vi "ground_station_control_only.vi"() -> ()   [LabVIEW 2017]
uses:
  <vilib>/Analysis/coordinate.llb/3D Cartesian Coordinate Rotation (Euler) (Array).vi
  <vilib>/Instr/_visa.llb/VISA Configure Serial Port (Instr).vi
  <vilib>/Analysis/NI_AALPro.lvlib
panel:
  out "read buffer":string
  in  "ZXZ":cluster{"phi":dbl, "theta":dbl, "psi":dbl} {"psi" min=0.0 max=6.28 step=0.01 format="%.2f"; "theta" min=0.0 max=3.14 step=0.01 format="%.2f"; "phi" min=0.0 max=6.28 step=0.001 format="%.2f"}
  out "时间差":u32 format="时间差 %.0f ms"
  out "外层":i32 format="外层循环 %.0f"
  out "String 4":string
  out "String 3":string
  in  "停止外层":bool
  out "Array":cluster{i32, i32, "read buffer":string}[](array[cluster])
  out "实际读取字节数":u32 format="实际读取的字节数 %.0f"
  out "内层":i32 format="内层循环 %.0f"
  in  "Z-":bool
  in  "Z+":bool
  in  "Y-":bool
  in  "Y+":bool
  in  "X-":bool
  in  "X+":bool
  out "error out 2":errorcluster
  out "String 2":string
  in  "Boolean":bool
  in  "VISA resource name":refnum<visa-resource-name>
  out "length":i32
  out "String":string
  out "error out":errorcluster
  in  "停止内层":bool
  in  "目标取向":dbl[][](array[numeric])
  in  "目标位置":dbl[](array[numeric]) step=0.1 format="%.1f"
  out "求解状态":i32
  out "关节角度":dbl[](array[numeric])
  in  "初始关节位置":dbl[][](array[numeric])
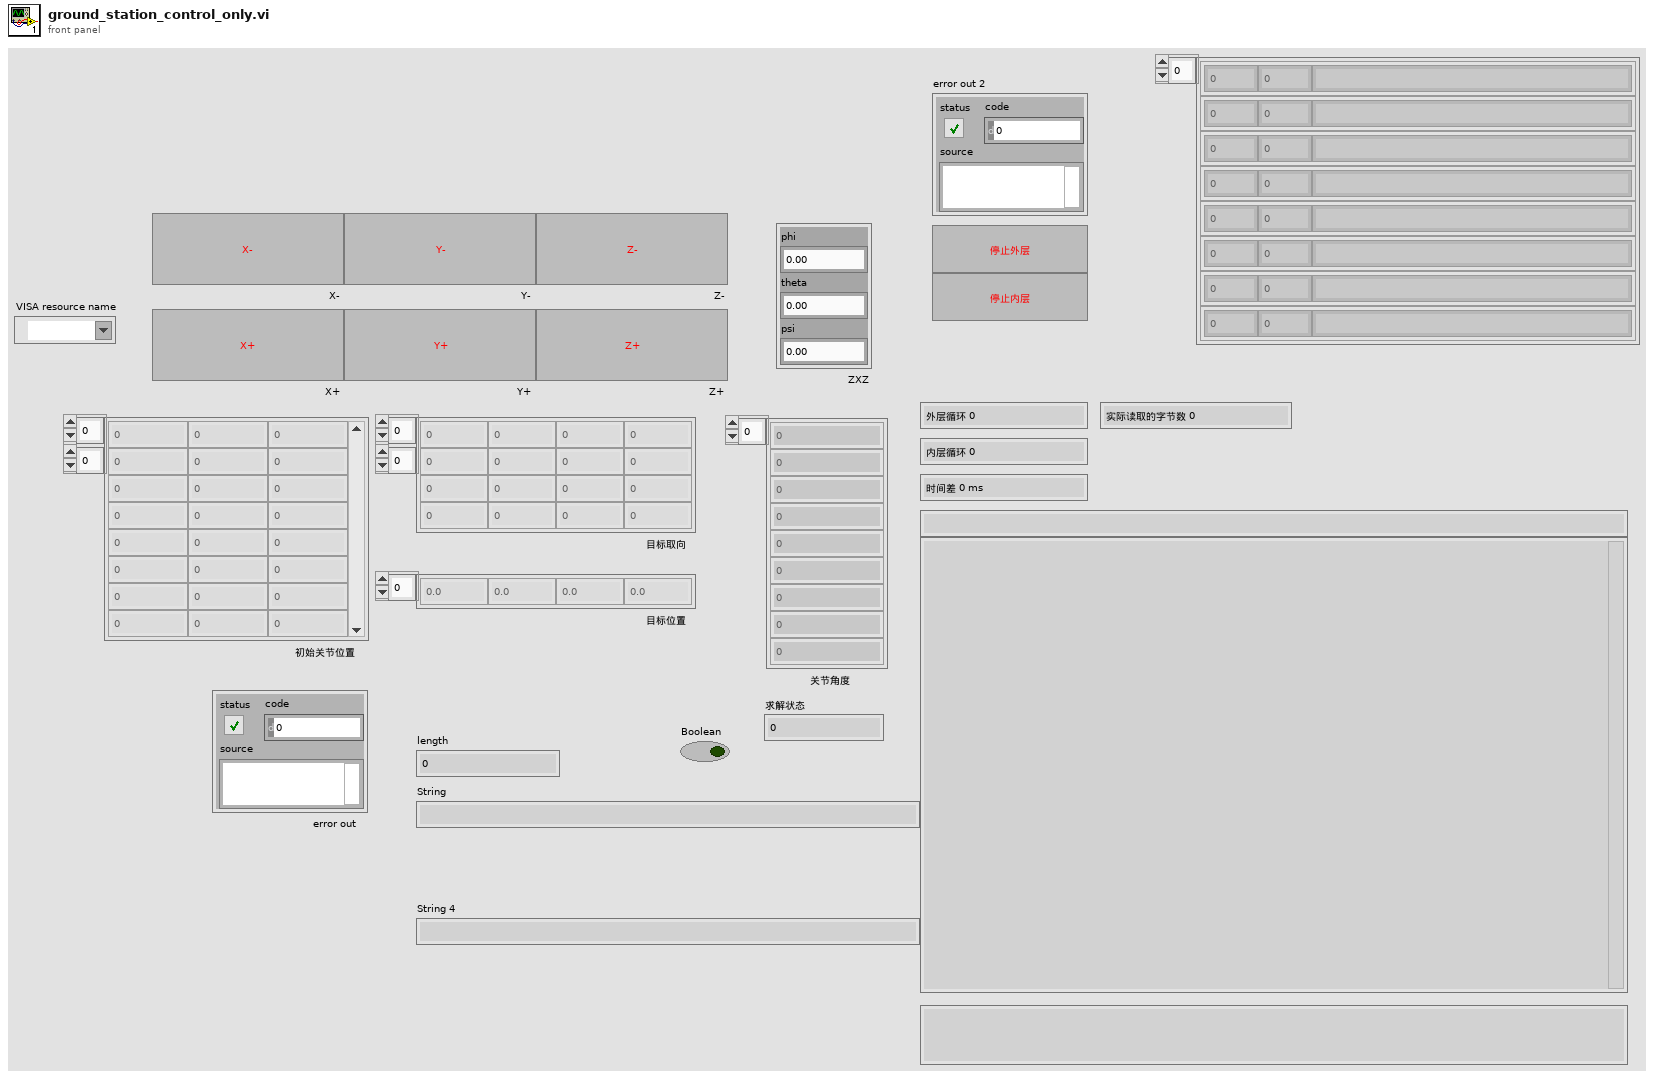
[diagram p1: front panel]
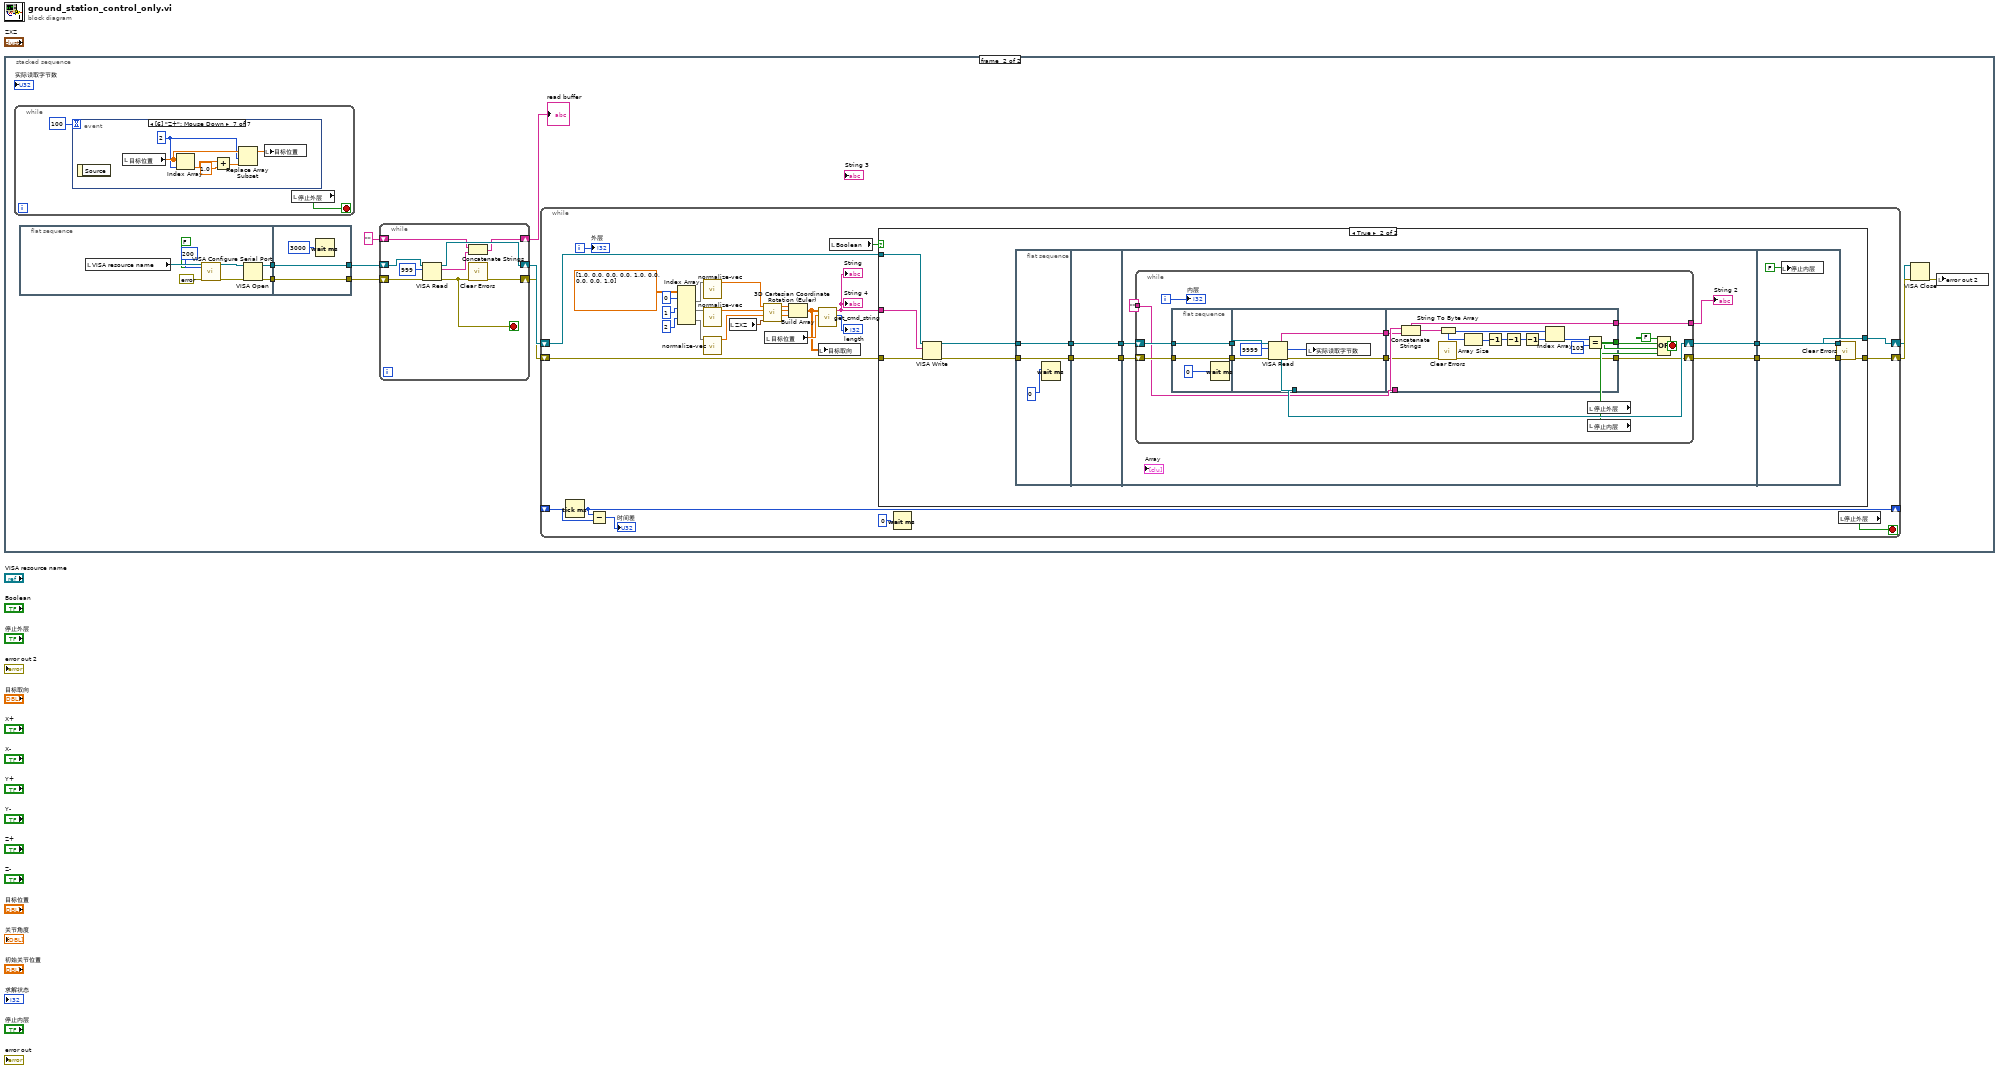
[diagram p0: block diagram]
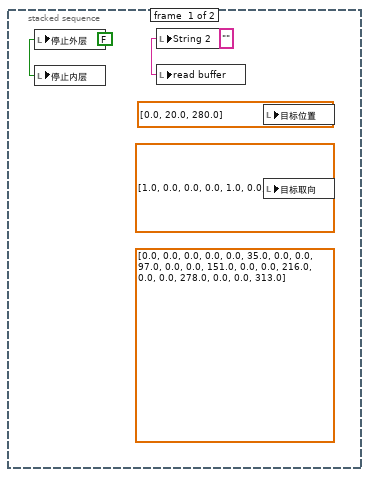
[diagram p2: hidden frame]
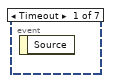
[diagram p4: hidden frame]
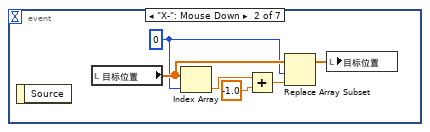
[diagram p5: hidden frame]
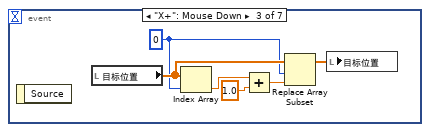
[diagram p6: hidden frame]
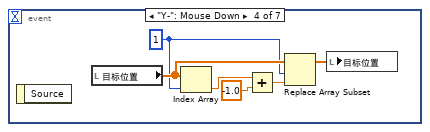
[diagram p7: hidden frame]
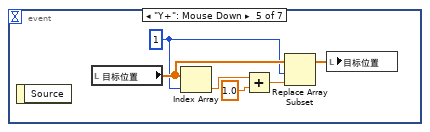
[diagram p8: hidden frame]
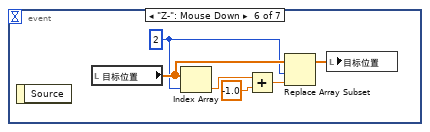
[diagram p9: hidden frame]
diagram:
  n1 = stacked-sequence {
    frame #0 {
      w1 = "" ("read buffer")
      w2 = FALSE ("stop")
      (unwired) dbl[][] [[0.0, 0.0, 0.0], [0.0, 0.0, 35.0], [0.0, 0.0, 97.0], [0.0, 0.0, 151.0], [0.0, 0.0, 216.0], [0.0, 0.0, 278.0], [0.0, 0.0, 313.0]] ("初始关节位置")
      n2 = local write "停止外层"(w2) -> ()
      n3 = local write "停止内层"(w2) -> ()
      n4 = local write "String 2"(w1) -> ()
      n5 = local write "read buffer"(w1) -> ()
      n6 = local write "目标位置"(dbl[] [0.0, 20.0, 280.0] ("初始关节位置")) -> ()
      n7 = local write "目标取向"(dbl[][] [[1.0, 0.0, 0.0], [0.0, 1.0, 0.0], [0.0, 0.0, 1.0]] ("初始关节位置")) -> ()
    }
    frame #1 {
      n8 = while {
        stop <- w134 stop-if-true
        n9 = event shown="[6] \"Z+\": Mouse Down" {
          selector: _ -> [_ _ _ _ _ _ _]
          dyn-events: _ -> [_ _ _ _ _ _ _]
          timeout: 100 -> [_ _ _ _ _ _ _]
          event Timeout {
            n10 = event-data() -> ()  [unwired: 1 in, 1 out]
          }
          event "X-": Mouse Down {
            w140 = 0 ("index")
            n11 = event-data() -> ()  [unwired: 1 in, 1 out]
            n12 = local read "目标位置"() -> (w141:dbl[])
            n13 = Index Array(array=w141, index=w140) -> (element=w139:dbl)
            n14 = Add(x=w139, y=-1.0 ("new element/subarray")) -> (x+y=w137:dbl)
            n15 = Replace Array Subset(array=w141, new element=w137, index=w140) -> (w136:dbl[])
            n16 = local write "目标位置"(w136) -> ()
          }
          event "X+": Mouse Down {
            w142 = 0 ("index")
            n17 = event-data() -> ()  [unwired: 1 in, 1 out]
            n18 = local read "目标位置"() -> (w147:dbl[])
            n19 = Index Array(array=w147, index=w142) -> (element=w146:dbl)
            n20 = Add(x=w146, y=1.0 ("new element/subarray")) -> (x+y=w145:dbl)
            n21 = Replace Array Subset(array=w147, new element=w145, index=w142) -> (w144:dbl[])
            n22 = local write "目标位置"(w144) -> ()
          }
          event "Y-": Mouse Down {
            w148 = 1 ("index")
            n23 = event-data() -> ()  [unwired: 1 in, 1 out]
            n24 = local read "目标位置"() -> (w153:dbl[])
            n25 = Index Array(array=w153, index=w148) -> (element=w152:dbl)
            n26 = Add(x=w152, y=-1.0 ("new element/subarray")) -> (x+y=w151:dbl)
            n27 = Replace Array Subset(array=w153, new element=w151, index=w148) -> (w150:dbl[])
            n28 = local write "目标位置"(w150) -> ()
          }
          event "Y+": Mouse Down {
            w154 = 1 ("index")
            n29 = event-data() -> ()  [unwired: 1 in, 1 out]
            n30 = local read "目标位置"() -> (w159:dbl[])
            n31 = Index Array(array=w159, index=w154) -> (element=w158:dbl)
            n32 = Add(x=w158, y=1.0 ("new element/subarray")) -> (x+y=w157:dbl)
            n33 = Replace Array Subset(array=w159, new element=w157, index=w154) -> (w156:dbl[])
            n34 = local write "目标位置"(w156) -> ()
          }
          event "Z-": Mouse Down {
            w160 = 2 ("index")
            n35 = event-data() -> ()  [unwired: 1 in, 1 out]
            n36 = local read "目标位置"() -> (w165:dbl[])
            n37 = Index Array(array=w165, index=w160) -> (element=w164:dbl)
            n38 = Add(x=w164, y=-1.0 ("new element/subarray")) -> (x+y=w163:dbl)
            n39 = Replace Array Subset(array=w165, new element=w163, index=w160) -> (w162:dbl[])
            n40 = local write "目标位置"(w162) -> ()
          }
          event "Z+": Mouse Down {
            w166 = 2 ("index")
            n41 = event-data() -> ()  [unwired: 1 in, 1 out]
            n42 = local read "目标位置"() -> (w171:dbl[])
            n43 = Index Array(array=w171, index=w166) -> (element=w170:dbl)
            n44 = Add(x=w170, y=1.0 ("new element/subarray")) -> (x+y=w169:dbl)
            n45 = Replace Array Subset(array=w171, new element=w169, index=w166) -> (w168:dbl[])
            n46 = local write "目标位置"(w168) -> ()
          }
        }
        n47 = local read "停止外层"() -> (w134:bool)
      }
      n48 = flat-sequence {
        tunnel: [w26] -> w12
        tunnel: [w25] -> w11
        tunnel: [w34] -> w10
        tunnel: [w35] -> w9
        tunnel: w12 -> [w35]
        tunnel: w11 -> [w34]
        frame #0 {
          n49 = local read "VISA resource name"() -> (w32:refnum<visa-resource-name>)
          n50 = call-poly "VISA Configure Serial Port"("VISA resource name"=w32, "timeout (10sec)"=u32 200, "Enable Termination\nChar (T)"=FALSE ("Enable Termination\nChar (T)"), "error in (no error)"=errorcluster {"status"=FALSE, "code"=0, "source"=""}) -> ("VISA resource name out"=w30:refnum<visa-resource-name>, "error out"=w31:errorcluster)  [unwired: 10 in]
          n51 = VISA Open(error in (no error)=w31, VISA resource name=w30) -> (VISA resource name=w26:refnum<visa-resource-name>, error out=w25:errorcluster)  [unwired: 3 in]
        }
        frame #1 {
          n52 = Wait (ms)(milliseconds to wait=u32 3000) -> ()  [unwired: 1 out]
        }
      }
      n53 = while {
        shift-right: [w18] -> w5
        shift-left: w10 -> [w23]
        shift-right: [w21] -> w6
        shift-left: w9 -> [w24]
        shift-right: [w19] -> w8
        shift-left: "" ("read buffer") -> [w20]
        stop <- w16 stop-if-true
        n54 = VISA Read(VISA resource name=w24, byte count=u32 999, error in (no error)=w23) -> (VISA resource name out=w21:refnum<visa-resource-name>, read buffer=w17:string, error out=w16:errorcluster)  [unwired: 1 out]
        n55 = Concatenate Strings(w20, w17) -> (w19:string)
        n56 = call <vilib>:"Clear Errors.vi"("error in (no error)"=w16) -> ("error out"=w18:errorcluster)  [unwired: 5 in, 1 out]
      }
      "read buffer" <- w8
      n57 = while {
        shift-right: [w60] -> w13
        shift-left: w6 -> [w59]
        shift-right: [w58] -> w14
        shift-left: w5 -> [w36]
        shift-right: [w52] -> _
        shift-left: _ -> [w54]
        i -> [w55]
        stop <- w57 stop-if-true
        n58 = Tick Count (ms)() -> (millisecond timer value=w52:u32)
        n59 = Subtract(x=w52, y=w54) -> (x-y=→"时间差":u32)
        n60 = Index Array(array=dbl[][] [[1.0, 0.0, 0.0], [0.0, 1.0, 0.0], [0.0, 0.0, 1.0]], index (row) #1=0 ("index (row)"), index (row) #2=1 ("index (row)"), index (row) #3=2 ("index (row)")) -> (element #1=w42:dbl[], element #2=w43:dbl[], element #3=w44:dbl[])  [unwired: 3 in]
        n61 = call "normalize-vec.vi"("Vec Input"=w42) -> ("Array Output"=w45:dbl[])  [unwired: 7 in, 3 out]
        n62 = call "normalize-vec.vi"("Vec Input"=w43) -> ("Array Output"=w46:dbl[])  [unwired: 7 in, 3 out]
        n63 = call "normalize-vec.vi"("Vec Input"=w44) -> ("Array Output"=w47:dbl[])  [unwired: 7 in, 3 out]
        n64 = local read "ZXZ"() -> (w51:cluster{"phi":dbl, "theta":dbl, "psi":dbl})
        n65 = call-poly <vilib>:"3D Cartesian Coordinate Rotation (Euler).vi"("Euler Angles"=w51, "Z"=w47, "Y"=w46, "X"=w45) -> ("Z Out"=w50:dbl[], "Y Out"=w49:dbl[], "X Out"=w48:dbl[])  [unwired: 4 in, 1 out]
        n66 = local read "目标位置"() -> (w64:dbl[])
        n67 = Build Array(w48, w49, w50) -> (w37:dbl[][])
        n68 = call "get_cmd_string.vi"("目标位置"=w64, "目标取向"=w37) -> ("length"=→"length":i32, "String"=w56:string)  [unwired: 8 in]
        "String" <- w56
        "String 4" <- w56
        n69 = local write "目标取向"(w37) -> ()
        n70 = local read "Boolean"() -> (w61:bool)
        n71 = case shown="True" w61 {
          tunnel: w56 -> [_ w80]
          tunnel: w59 -> [w66 w79]
          tunnel: w36 -> [w65 w78]
          tunnel: [w65 w76] -> w58
          tunnel: [w66 w74] -> w60
          frame False {
          }
          frame True {
            n72 = VISA Write(VISA resource name=w79, write buffer=w80, error in (no error)=w78) -> (VISA resource name out=w75:refnum<visa-resource-name>, error out=w67:errorcluster)  [unwired: 1 out]
            n73 = flat-sequence {
              tunnel: w75 -> [w82]
              tunnel: w67 -> [w83]
              tunnel: [w83] -> w71
              tunnel: [w82] -> w70
              tunnel: [w85] -> w73
              tunnel: [w84] -> w72
              tunnel: w71 -> [w85]
              tunnel: w70 -> [w84]
              tunnel: w73 -> [w90]
              tunnel: w72 -> [w89]
              tunnel: [w91] -> w69
              tunnel: [w88] -> w68
              tunnel: [w132] -> w74
              tunnel: [w133] -> w77
              tunnel: w69 -> [w133]
              tunnel: w68 -> [w132]
              frame #0 {
                n74 = Wait (ms)(milliseconds to wait=u32 0) -> ()  [unwired: 1 out]
              }
              frame #1 {
              }
              frame #2 {
                n75 = while {
                  shift-right: [w103] -> w91
                  shift-left: w90 -> [w107]
                  shift-right: [w105] -> w88
                  shift-left: w89 -> [w106]
                  tunnel: "" -> [w95]
                  tunnel: [w93] -> w86
                  i -> [w96]
                  stop <- w102 stop-if-true
                  n76 = flat-sequence {
                    tunnel: w106 -> [w109]
                    tunnel: w107 -> [w110]
                    tunnel: [w110] -> w99
                    tunnel: [w109] -> w98
                    tunnel: [w115] -> w105
                    tunnel: [w113] -> w100
                    tunnel: w99 -> [w117]
                    tunnel: w98 -> [w116]
                    tunnel: [w111] -> w94
                    tunnel: [w118] -> w103
                    tunnel: w100 -> [w119]
                    tunnel: w95 -> [w128]
                    tunnel: w94 -> [w127]
                    tunnel: [w125] -> w93
                    tunnel: [w121] -> w92
                    frame #0 {
                      n77 = Wait (ms)(milliseconds to wait=u32 0) -> ()  [unwired: 1 out]
                    }
                    frame #1 {
                      n78 = VISA Read(VISA resource name=w116, byte count=u32 9999, error in (no error)=w117) -> (VISA resource name out=w115:refnum<visa-resource-name>, read buffer=w111:string, return count=w112:u32, error out=w113:errorcluster)
                      n79 = local write "实际读取字节数"(w112) -> ()
                    }
                    frame #2 {
                      n80 = Concatenate Strings(w128, w127) -> (w125:string)
                      n81 = call <vilib>:"Clear Errors.vi"("error in (no error)"=w119) -> ("error out"=w118:errorcluster)  [unwired: 5 in, 1 out]
                      n82 = String To Byte Array(string=w125) -> (unsigned byte array=w126:u8[])
                      n83 = Array Size(array=w126) -> (size(s)=w129:i32)
                      n84 = Decrement(x=w129) -> (x-1=w130:i32)
                      n85 = Decrement(x=w130) -> (x-1=w123:i32)
                      n86 = Decrement(x=w123) -> (x-1=w120:i32)
                      n87 = Index Array(array=w126, index=w120) -> (element=w124:u8)
                      n88 = Equal?(x=w124, y=103) -> (x = y?=w121:bool)
                    }
                  }
                  n89 = local read "停止外层"() -> (w101:bool)
                  n90 = local read "停止内层"() -> (w104:bool)
                  n91 = Compound Arithmetic op=OR(FALSE ("value"), w104, w92, w101) -> (w102:bool)
                  "内层" <- w96
                }
                "String 2" <- w86
              }
              frame #3 {
                n92 = local write "停止内层"(FALSE ("停止")) -> ()
              }
            }
            n93 = call <vilib>:"Clear Errors.vi"("error in (no error)"=w77) -> ("error out"=w76:errorcluster)  [unwired: 5 in, 1 out]
          }
        }
        n94 = Wait (ms)(milliseconds to wait=u32 0) -> ()  [unwired: 1 out]
        n95 = local read "停止外层"() -> (w57:bool)
        "外层" <- w55
      }
      n96 = VISA Close(VISA resource name=w13, error in (no error)=w14) -> (error out=w15:errorcluster)
      n97 = local write "error out 2"(w15) -> ()
    }
  }
